vi "checkFinishEnemyPossessionAtOurField.vi"(8 "error in (no error)":errorcluster, 9 "last command_interpreted":T1, 10 "Game":refnum<class "Game.lvclass">, 11 "EnemyPossessionAtOurFieldPlay in":refnum<class "EnemyPossessionAtOurFieldPlay.lvclass">) -> (0 "error out":errorcluster, 2 "Boolean":bool, 3 "EnemyPossessionAtOurFieldPlay out":refnum<class "EnemyPossessionAtOurFieldPlay.lvclass">)   [LabVIEW 2023, in "EnemyPossessionAtOurFieldPlay.lvclass"]
uses:
  EnemyPossessionAtOurFieldPlay.lvclass
  Game_class/Game.lvclass
  Referee_class/command_interpreted.ctl
  Game_class/Game.lvclass/Game.ctl
  Referee_class/Referee.lvclass/Referee.ctl
  Events_class/Events.lvclass/Events.ctl
  Object_class/Object.lvclass/Object.ctl
  Game_class/Read Referee.vi
  Game_class/Read EventsRef.vi
  Game_class/Read BallRef.vi
  Object_class/Read x.vi
  Events_class/Read ball_out.vi
  Events_class/Read enemy_ball_possesion.vi
  Referee_class/Read command_interpreted.vi
  Ball_class/Ball.lvclass
  Referee_class/Referee.lvclass
  Events_class/Events.lvclass
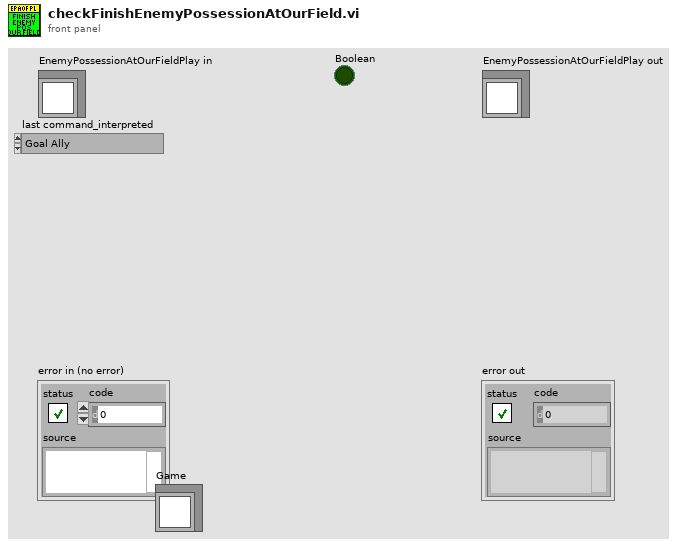
[diagram p1: front panel]
types:
  T1 = typedef "command_interpreted.ctl" = enum16{"Goal Ally", "Goal Enemy", "Ball Placement Enemy", "Ball Placement Ally", "Normal Half Time", "Extra Time  Break", "Extra Half Time", "None", "Post Game", "PKA Normal Start", "Prepare Kickoff Ally", "PKE Normal Start", "Prepare Kickoff Enemy", "Force Start", "Halt", "Timeout", "Prepare Penalty Ally", "Prepare Penalty Enemy", "PPA NormalStart", "PPE Normal Start", "Indirect Free Ally", "Direct Free Enemy", "Direct Free Ally", "Indirect Free Enemy", "Stop"}
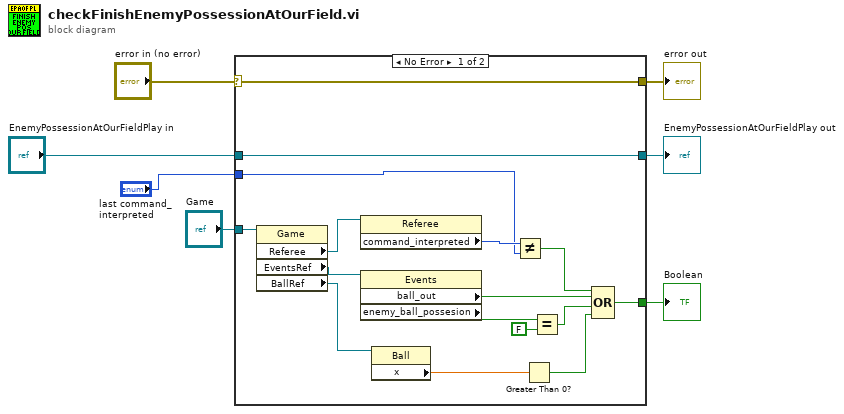
[diagram p0: block diagram]
diagram:
  n1 = case shown="No Error" "error in (no error)" {
    selector: "error in (no error)" -> [w22 w25]
    tunnel: [w22 w25] -> w6
    tunnel: [w23 w24] -> w4
    tunnel: "EnemyPossessionAtOurFieldPlay in" -> [w23 w24]
    tunnel: "Game" -> [w12 _]
    tunnel: [w9 _] -> w2
    tunnel: "last command_interpreted" -> [w8 _]
    frame No Error {
      n2 = property class="Game"(reference=w12) -> ("Referee"=w21:refnum<class "Referee.lvclass">, "EventsRef"=w19:refnum<class "Events.lvclass">, "BallRef"=w14:refnum<class "Ball.lvclass">)  [unwired: 1 in, 2 out]
      n3 = property class="Referee"(reference=w21) -> ("command_interpreted"=w20:T1)  [unwired: 1 in, 2 out]
      n4 = property class="Events"(reference=w19) -> ("ball_out"=w17:bool, "enemy_ball_possesion"=w16:bool)  [unwired: 1 in, 2 out]
      n5 = property class="Ball"(reference=w14) -> ("x"=w13:dbl)  [unwired: 1 in, 2 out]
      n6 = Not Equal?(x=w20, y=w8) -> (x != y?=w18:bool)
      n7 = Greater Than 0?(x=w13) -> (x > 0?=w10:bool)
      n8 = Equal?(x=w16, y=FALSE) -> (x = y?=w15:bool)
      n9 = Compound Arithmetic op=OR(w18, w17, w15, w10) -> (w9:bool)
    }
    frame Error {
    }
  }
  "error out" <- w6
  "EnemyPossessionAtOurFieldPlay out" <- w4
  "Boolean" <- w2
